vi "Host - Configuration to command.vi"(6 "Operation Index":i32, 7 "Async":T1={"Interface"="Async", "Interface Data"={"Command"="Configure", "SubCmd"="Async", "Data"=[{"Port"="com2", "Minor Frame Freq"=20, "Minor Frame Count"=1, "Frame Info"=[{"Frame ID"=1, "Message Info"=[{"Message"=[1, 2, 3, 4], "Message Name"="m1"}]}], "Sensor Type"=0, "OIM Address"=0}]}} {"Interface Data"."Data"."Minor Frame Count" min=5 max=8 step=1}, 8 "error in":errorcluster, 9 "AI":T9={"Interface"="AIO", "Interface Data"={"Command"="Configure", "SubCmd"="AI", "Data"=[{"Channel"="Mod1/ai0", "Min Value"=-5.0, "Max Value"=5.0, "Type"="Voltage", "Terminal Configure"=10083, "Dynamic"=0, "Dyn Type"="", "Data"=[], "File Name"="", "Column"=0, "Frequency"=0.0}, {"Channel"="Mod1/ai1", "Min Value"=-5.0, "Max Value"=5.0, "Type"="Voltage", "Terminal Configure"=10083, "Dynamic"=0, "Dyn Type"="", "Data"=[], "File Name"="", "Column"=0, "Frequency"=0.0}], "Timing"={"samples per channel"=4, "sample mode"=10123, "Sampling Rate"=2.0}}} {"Interface Data"."Timing"."sample mode" items=["Finite Samples"=10178, "Continuous Samples"=10123, "Hardware Timed Single Point"=12522]}, 10 "DO":T6={"Interface"="DIO", "Interface Data"={"Command"="Configure", "SubCmd"="DO", "Frequency"=20, "Data"=[{"Channel"="Mod2/port0/line0", "Data"=[], "Identification Name"=""}, {"Channel"="Mod2/port0/line1", "Data"=[], "Identification Name"=""}, {"Channel"="Mod2/port0/line2", "Data"=[], "Identification Name"=""}, {"Channel"="Mod2/port0/line3", "Data"=[], "Identification Name"=""}]}}, 11 "DI":T6={"Interface"="DIO", "Interface Data"={"Command"="Configure", "SubCmd"="DI", "Frequency"=20, "Data"=[{"Channel"="Mod2/port0/line0", "Data"=[], "Identification Name"=""}, {"Channel"="Mod2/port0/line1", "Data"=[], "Identification Name"=""}, {"Channel"="Mod2/port0/line2", "Data"=[], "Identification Name"=""}, {"Channel"="Mod2/port0/line3", "Data"=[], "Identification Name"=""}]}}) -> (0 "error out":errorcluster, 3 "Command Data":string[](array[string]))   [LabVIEW 2024]
uses:
  Analog Output/Controls/AO JSON Data Cluster.ctl
  Analog Output/Controls/AO Interface Data Cluster.ctl
  Analog Output/Controls/AO Channel Configuration Cluster.ctl
  Analog Output/Controls/AO Timing Cluster.ctl
  Digital Output/Controls/DIO Configuration cluster.ctl
  Digital Output/Controls/DIO Interface Data.ctl
  Digital Output/SubVIs/Digital Dynamic Cluster.ctl
  Async JSON Cluster.ctl
  Async Interface Data Cluster.ctl
  Async Serial/Controls/Async Serial Configuration Cluster.ctl
  Async Serial/Controls/Async Frame Info Cluster.ctl
  Async Serial/Controls/Async Message Info Cluster.ctl
  <vilib>/Utility/error.llb/Trim Whitespace One-Sided.vi
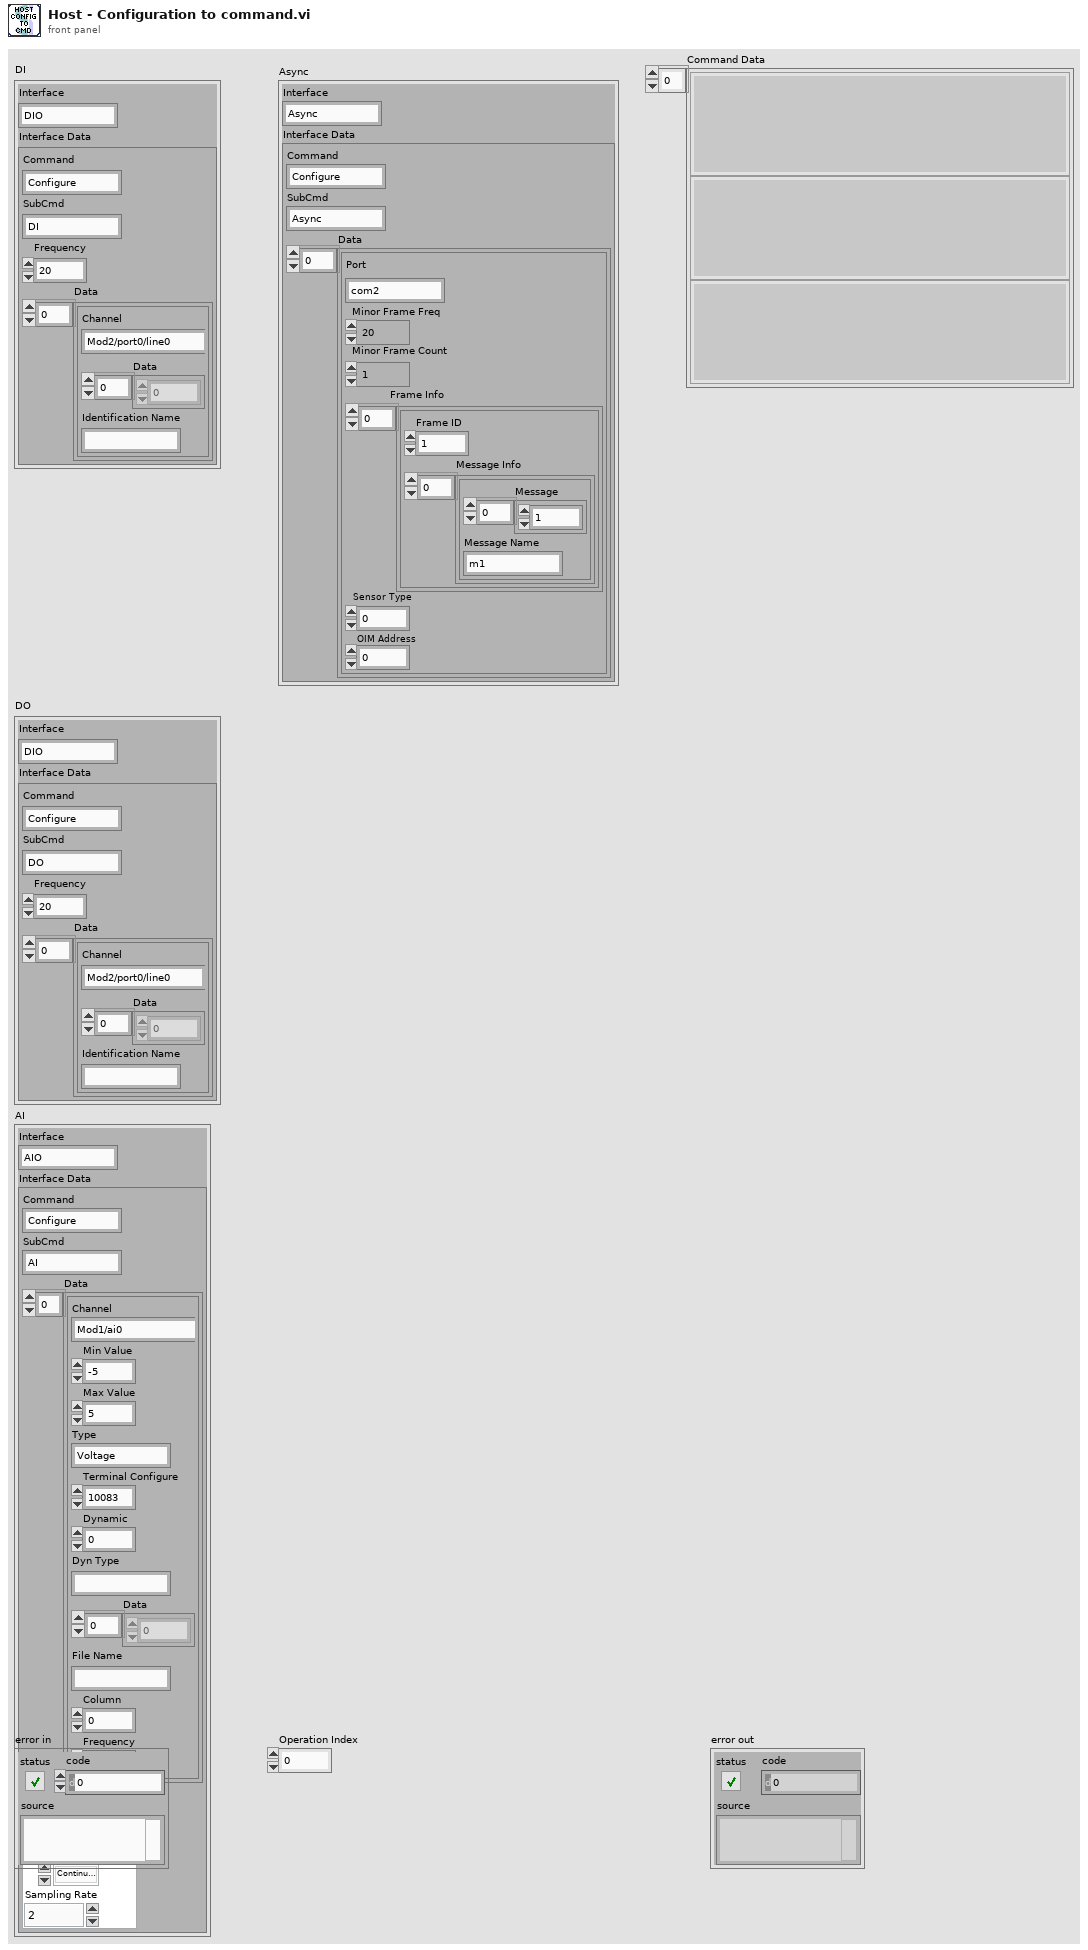
[diagram p1: front panel]
types:
  T1 = typedef "Async JSON Cluster.ctl" = cluster{"Interface":string, "Interface Data":T2}
  T2 = typedef "Async Interface Data Cluster.ctl" = cluster{"Command":string, "SubCmd":string, "Data":T3[]}
  T3 = typedef "Async Serial Configuration Cluster.ctl" = cluster{"Port":string, "Minor Frame Freq":u16, "Minor Frame Count":u16, "Frame Info":T4[], "Sensor Type":u16, "OIM Address":u16}
  T4 = typedef "Async Frame Info Cluster.ctl" = cluster{"Frame ID":u16, "Message Info":T5[]}
  T5 = typedef "Async Message Info Cluster.ctl" = cluster{"Message":u8[], "Message Name":string}
  T6 = typedef "DIO Configuration cluster.ctl" = cluster{"Interface":string, "Interface Data":T7}
  T7 = typedef "DIO Interface Data.ctl" = cluster{"Command":string, "SubCmd":string, "Frequency":u16, "Data":T8[]}
  T8 = typedef "Digital Dynamic Cluster.ctl" = cluster{"Channel":string, "Data":u8[], "Identification Name":string}
  T9 = typedef "AO JSON Data Cluster.ctl" = cluster{"Interface":string, "Interface Data":T10}
  T10 = typedef "AO Interface Data Cluster.ctl" = cluster{"Command":string, "SubCmd":string, "Data":T11[], "Timing":T12}
  T11 = typedef "AO Channel Configuration Cluster.ctl" = cluster{"Channel":string, "Min Value":dbl, "Max Value":dbl, "Type":string, "Terminal Configure":u16, "Dynamic":u8, "Dyn Type":string, "Data":dbl[], "File Name":string, "Column":i32, "Frequency":dbl}
  T12 = typedef "AO Timing Cluster.ctl" = cluster{"samples per channel":i32, "sample mode":i32, "Sampling Rate":dbl}
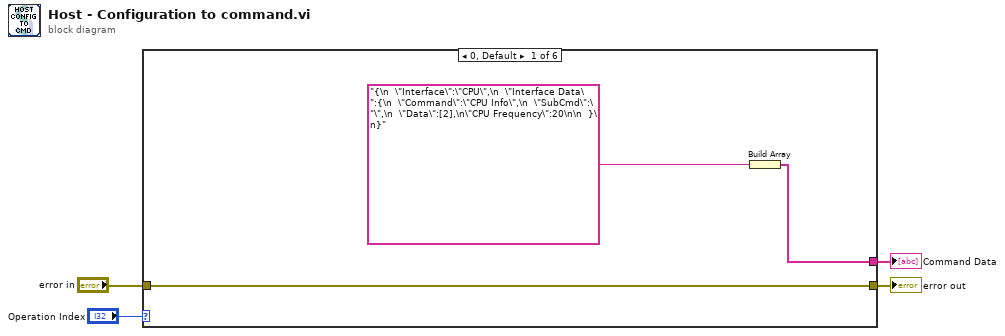
[diagram p0: block diagram]
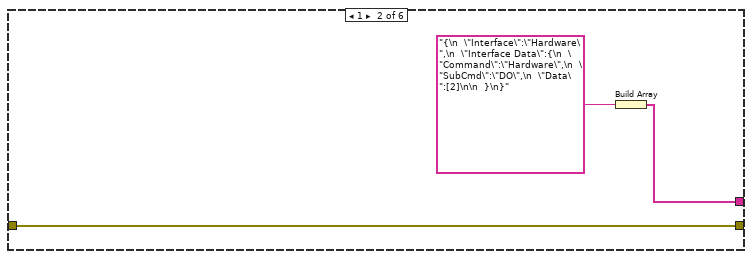
[diagram p2: hidden frame]
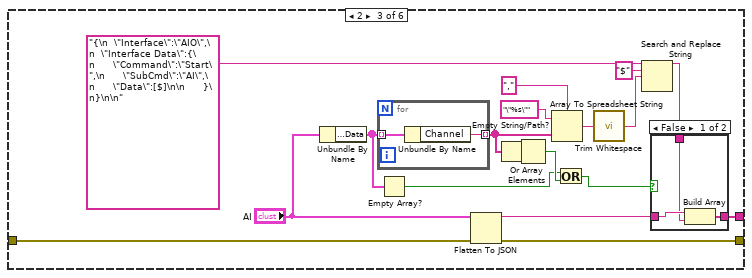
[diagram p3: hidden frame]
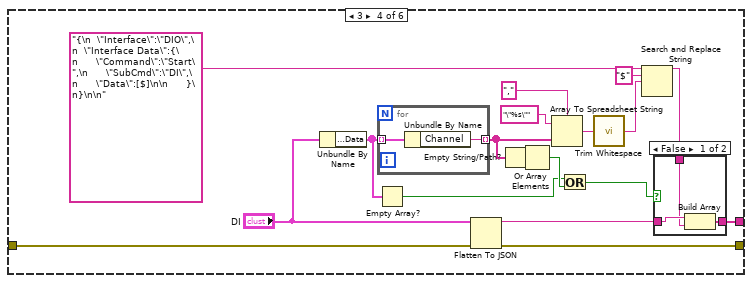
[diagram p5: hidden frame]
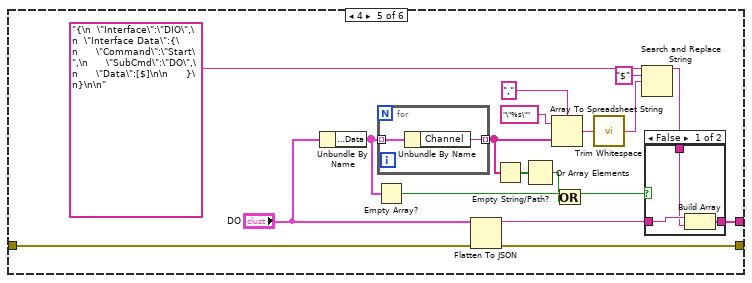
[diagram p7: hidden frame]
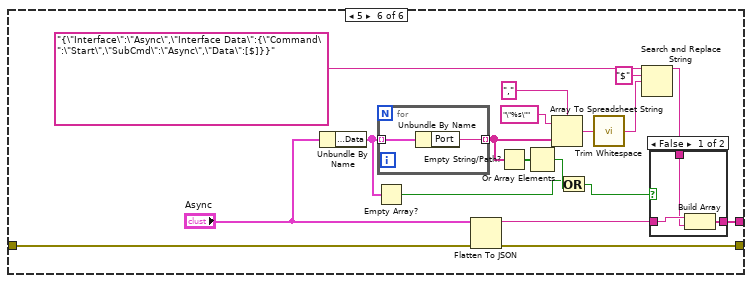
[diagram p9: hidden frame]
diagram:
  n1 = case shown="0, Default" "Operation Index" {
    tunnel: "error in" -> [w6 w8 w28 w51 w74 w97]
    tunnel: [w6 w8 w27 w50 w73 w96] -> w4
    tunnel: [w7 w9 w17 w41 w64 w87] -> w3
    frame 0, Default {
      n2 = Build Array("{\n  \"Interface\":\"CPU\",\n  \"Interface Data\":{\n  \"Command\":\"CPU Info\",\n  \"SubCmd\":\"\",\n  \"Data\":[2],\n\"CPU Frequency\":20\n\n  }\n}" ("Data 2")) -> (w7:string[])
    }
    frame 1 {
      n3 = Build Array("{\n  \"Interface\":\"Hardware\",\n  \"Interface Data\":{\n  \"Command\":\"Hardware\",\n  \"SubCmd\":\"DO\",\n  \"Data\":[2]\n\n  }\n}" ("Data 2")) -> (w9:string[])
    }
    frame 2 {
      n4 = Unbundle By Name("AI") -> ("Interface Data.Data"=w16:T11[])
      n5 = for {
        tunnel: w16 -> [w33] mode=indexing
        tunnel: [w32] -> w13 mode=indexing
        n6 = Unbundle By Name(w33) -> ("Channel"=w32:string)
      }
      n7 = Empty Array?(array=w16) -> (empty?=w12:bool)
      n8 = Flatten To JSON(anything="AI", error in (no error)=w28) -> (JSON string=w22:string, 11:w27:errorcluster)  [unwired: 1 in]
      n9 = Empty String/Path?(string/path=w13) -> (empty?=w14:bool[])
      n10 = Or Array Elements(Boolean array=w14) -> (logical OR=w15:bool)
      n11 = Array To Spreadsheet String(delimiter (Tab)=",", array=w13, 3:"\"%s\"" ("format string")) -> (spreadsheet string=w24:string)
      n12 = Or(x=w12, y=w15) -> (x .or. y?=w11:bool)
      n13 = call <vilib>:"Trim Whitespace.vi"("string"=w24) -> ("trimmed string"=w19:string)  [unwired: 1 in]
      n14 = Search and Replace String(input string="{\n  \"Interface\":\"AIO\",\n  \"Interface Data\":{\n      \"Command\":\"Start\",\n      \"SubCmd\":\"AI\",\n      \"Data\":[$]\n\n      }\n}\n\n" ("AI_start"), search string="$", replace string=w19) -> (result string=w18:string)  [unwired: 5 in, 3 out]
      n15 = case shown="False" w11 {
        tunnel: w22 -> [w31 _]
        tunnel: w18 -> [w30 _]
        tunnel: [w29 _] -> w17
        frame False {
          n16 = Build Array(w31, w30) -> (w29:string[])
        }
        frame True {
        }
      }
    }
    frame 3 {
      n17 = Unbundle By Name("DI") -> ("Interface Data.Data"=w39:T8[])
      n18 = Empty Array?(array=w39) -> (empty?=w35:bool)
      n19 = for {
        tunnel: w39 -> [w56] mode=indexing
        tunnel: [w55] -> w36 mode=indexing
        n20 = Unbundle By Name(w56) -> ("Channel"=w55:string)
      }
      n21 = Flatten To JSON(anything="DI", error in (no error)=w51) -> (JSON string=w46:string, 11:w50:errorcluster)  [unwired: 1 in]
      n22 = Empty String/Path?(string/path=w36) -> (empty?=w38:bool[])
      n23 = Or Array Elements(Boolean array=w38) -> (logical OR=w37:bool)
      n24 = Array To Spreadsheet String(delimiter (Tab)=",", array=w36, 3:"\"%s\"" ("format string")) -> (spreadsheet string=w47:string)
      n25 = Or(x=w35, y=w37) -> (x .or. y?=w34:bool)
      n26 = call <vilib>:"Trim Whitespace.vi"("string"=w47) -> ("trimmed string"=w43:string)  [unwired: 1 in]
      n27 = Search and Replace String(input string="{\n  \"Interface\":\"DIO\",\n  \"Interface Data\":{\n      \"Command\":\"Start\",\n      \"SubCmd\":\"DI\",\n      \"Data\":[$]\n\n      }\n}\n\n" ("AI_start"), search string="$", replace string=w43) -> (result string=w42:string)  [unwired: 5 in, 3 out]
      n28 = case shown="False" w34 {
        tunnel: w46 -> [w54 _]
        tunnel: w42 -> [w53 _]
        tunnel: [w52 _] -> w41
        frame False {
          n29 = Build Array(w54, w53) -> (w52:string[])
        }
        frame True {
        }
      }
    }
    frame 4 {
      n30 = Unbundle By Name("DO") -> ("Interface Data.Data"=w62:T8[])
      n31 = Empty Array?(array=w62) -> (empty?=w61:bool)
      n32 = for {
        tunnel: w62 -> [w79] mode=indexing
        tunnel: [w78] -> w60 mode=indexing
        n33 = Unbundle By Name(w79) -> ("Channel"=w78:string)
      }
      n34 = Flatten To JSON(anything="DO", error in (no error)=w74) -> (JSON string=w69:string, 11:w73:errorcluster)  [unwired: 1 in]
      n35 = Empty String/Path?(string/path=w60) -> (empty?=w58:bool[])
      n36 = Or Array Elements(Boolean array=w58) -> (logical OR=w57:bool)
      n37 = Array To Spreadsheet String(delimiter (Tab)=",", array=w60, 3:"\"%s\"" ("format string")) -> (spreadsheet string=w70:string)
      n38 = Or(x=w61, y=w57) -> (x .or. y?=w59:bool)
      n39 = call <vilib>:"Trim Whitespace.vi"("string"=w70) -> ("trimmed string"=w66:string)  [unwired: 1 in]
      n40 = Search and Replace String(input string="{\n  \"Interface\":\"DIO\",\n  \"Interface Data\":{\n      \"Command\":\"Start\",\n      \"SubCmd\":\"DO\",\n      \"Data\":[$]\n\n      }\n}\n\n" ("AI_start"), search string="$", replace string=w66) -> (result string=w65:string)  [unwired: 5 in, 3 out]
      n41 = case shown="False" w59 {
        tunnel: w69 -> [w77 _]
        tunnel: w65 -> [w76 _]
        tunnel: [w75 _] -> w64
        frame False {
          n42 = Build Array(w77, w76) -> (w75:string[])
        }
        frame True {
        }
      }
    }
    frame 5 {
      n43 = Unbundle By Name("Async") -> ("Interface Data.Data"=w85:T3[])
      n44 = Empty Array?(array=w85) -> (empty?=w81:bool)
      n45 = for {
        tunnel: w85 -> [w102] mode=indexing
        tunnel: [w101] -> w82 mode=indexing
        n46 = Unbundle By Name(w102) -> ("Port"=w101:string)
      }
      n47 = Flatten To JSON(anything="Async", error in (no error)=w97) -> (JSON string=w92:string, 11:w96:errorcluster)  [unwired: 1 in]
      n48 = Empty String/Path?(string/path=w82) -> (empty?=w84:bool[])
      n49 = Or Array Elements(Boolean array=w84) -> (logical OR=w83:bool)
      n50 = Array To Spreadsheet String(delimiter (Tab)=",", array=w82, 3:"\"%s\"" ("format string")) -> (spreadsheet string=w93:string)
      n51 = Or(x=w81, y=w83) -> (x .or. y?=w80:bool)
      n52 = call <vilib>:"Trim Whitespace.vi"("string"=w93) -> ("trimmed string"=w89:string)  [unwired: 1 in]
      n53 = Search and Replace String(input string="{\"Interface\":\"Async\",\"Interface Data\":{\"Command\":\"Start\",\"SubCmd\":\"Async\",\"Data\":[$]}}" ("AI_start"), search string="$", replace string=w89) -> (result string=w88:string)  [unwired: 5 in, 3 out]
      n54 = case shown="False" w80 {
        tunnel: w92 -> [w100 _]
        tunnel: w88 -> [w99 _]
        tunnel: [w98 _] -> w87
        frame False {
          n55 = Build Array(w100, w99) -> (w98:string[])
        }
        frame True {
        }
      }
    }
  }
  "error out" <- w4
  "Command Data" <- w3
